vi "Vision - Get Images for Sections.vi"(6 "Sections":T1[](array[typedef]), 8 "error in (no error)":errorcluster, 9 "Filename _L":string[](array[string]), 10 "Image Distances _L":dbl[](array[numeric]), 11 "Image Folder in":path) -> (0 "error out":errorcluster, 2 "Image Distances":dbl[](array[numeric]), 3 "Image Paths":path[](array[path]))   [LabVIEW 2024]
uses:
  Controls/Vision - Section.ctl
  Buttons/Bin.ctl
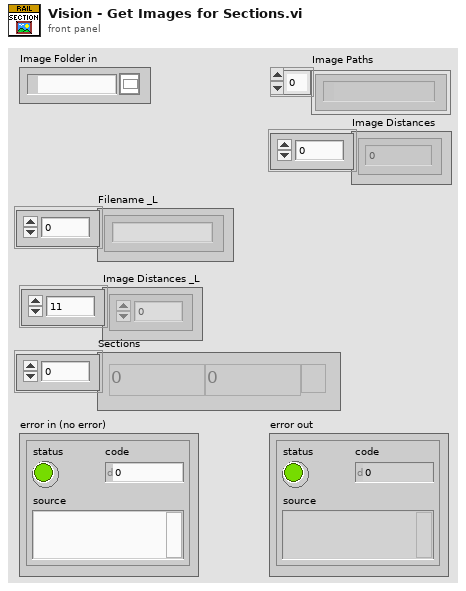
[diagram p1: front panel]
types:
  T1 = typedef "Vision - Section.ctl" = cluster{"From":dbl, "To":dbl, "Discard":T2}
  T2 = typedef "Bin.ctl" = bool
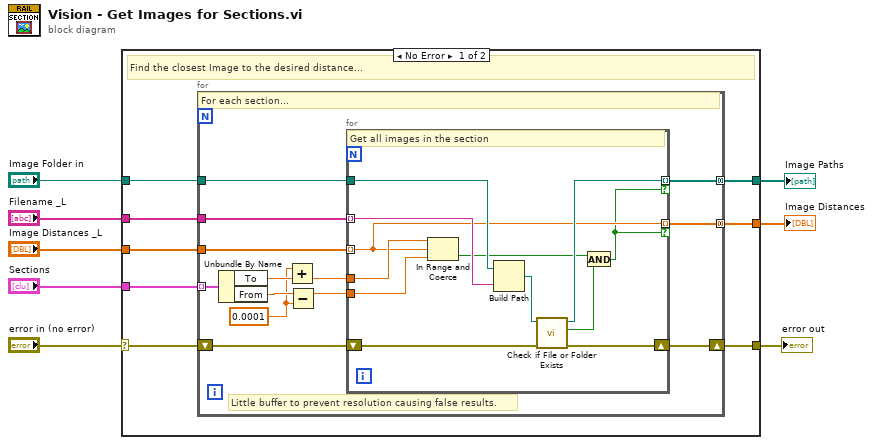
[diagram p0: block diagram]
diagram:
  n1 = case shown="No Error" "error in (no error)" {
    selector: "error in (no error)" -> [w13 w42]
    tunnel: "Image Distances _L" -> [w16 _]
    tunnel: "Filename _L" -> [w15 _]
    tunnel: "Image Folder in" -> [w14 _]
    tunnel: [w12 w42] -> w8
    tunnel: "Sections" -> [w10 _]
    tunnel: [w11 _] -> w2
    tunnel: [w9 _] -> w1
    frame No Error {
      # "Find the closest Image to the desired distance..."
      n2 = for {
        tunnel: w16 -> [w29]
        tunnel: w15 -> [w28]
        shift-right: [w25] -> w12
        shift-left: w13 -> [w26]
        tunnel: w14 -> [w27]
        tunnel: [w24] -> w11 mode=concatenating
        tunnel: w10 -> [w23] mode=indexing
        tunnel: [w20] -> w9 mode=concatenating
        w17 = 0.0001 ("y")
        # "Little buffer to prevent resolution causing false results."
        # "For each section..."
        n3 = Unbundle By Name(w23) -> ("To"=w22:dbl, "From"=w21:dbl)
        n4 = Add(x=w17, y=w22) -> (x+y=w19:dbl)
        n5 = Subtract(x=w21, y=w17) -> (x-y=w18:dbl)
        n6 = for {
          tunnel: w29 -> [w31] mode=indexing
          tunnel: w28 -> [w35] mode=indexing
          shift-right: [w39] -> w25
          shift-left: w26 -> [w40]
          tunnel: w27 -> [w41]
          tunnel: [w37] -> w24 mode=indexing if=w30
          tunnel: w19 -> [w34]
          tunnel: w18 -> [w33]
          tunnel: [w31] -> w20 mode=indexing if=w30
          # "Get all images in the section"
          n7 = In Range and Coerce(upper limit=w34, x=w31, lower limit=w33) -> (In Range?=w32:bool)  [unwired: 1 out]
          n8 = Build Path(base path=w41, name or relative path=w35) -> (appended path=w38:path)
          n9 = call <vilib>:"Check if File or Folder Exists.vi"("error in (no error)"=w40, "path"=w38) -> ("error out"=w39:errorcluster, "file or folder exists?"=w36:bool, "dup path"=w37:path)  [unwired: 7 in]
          n10 = And(x=w32, y=w36) -> (x .and. y?=w30:bool)
        }
      }
    }
    frame Error {
    }
  }
  "error out" <- w8
  "Image Paths" <- w2
  "Image Distances" <- w1
